vi "Mashina_podyehala.vi"() -> ()   [LabVIEW 2019]
panel:
  in  "Mashina podyehala":bool
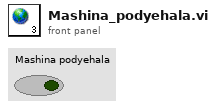
[diagram p1: front panel]
diagram:
